vi "PH_VacuumControl.contents.vi"   [LabVIEW 2014, in "PH_VacuumControl.lvlib"]
doc: "This class reads out an AGCxxx vacuum controller. Also the unit can be set. \n\nThis class is part of the PHELIX device layer."
uses:
  PH_VacuumControl.lvlib
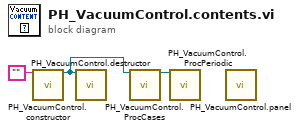
[diagram p0: block diagram]
diagram:
  n1 = call "PH_VacuumControl.constructor.vi"("name"="") -> ("i ref out"=w1:refnum<vi>)  [unwired: 16 in, 2 out]
  n2 = call "PH_VacuumControl.destructor.vi"("i ref in"=w1) -> ()  [unwired: 18 in, 1 out]
  n3 = call "PH_VacuumControl.ProcCases.vi"("i ref in"=w1) -> ("i ref out"=w2:refnum<vi>)  [unwired: 16 in, 2 out]
  n4 = call "PH_VacuumControl.ProcPeriodic.vi"("i ref in"=w2) -> ()  [unwired: 16 in, 3 out]
  n5 = call "PH_VacuumControl.panel.vi"() -> ()  [unwired: 19 in, 1 out]
